vi "StopDrive.vi"(8 "Drive Params":T1={"Omni"=TRUE, "Low Gear"=TRUE}) -> ()   [LabVIEW 2013]
uses:
  AutoDriveParams.ctl
  Drivetrain/Drivetrain Control.ctl
  Drivetrain/DT Mode.ctl
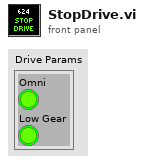
[diagram p1: front panel]
types:
  T1 = typedef "AutoDriveParams.ctl" = cluster{"Omni":bool, "Low Gear":bool}
  T2 = typedef "Drivetrain Control.ctl" = cluster{"axis 1 (x)":dbl, "axis 2 (y)":dbl, "Mode":T3, "heading target":dbl, "steer axis":dbl, "omni?":bool, "Low Gear?":bool, "distance target":cluster{"x":dbl, "y":dbl}, "PID Params":cluster{"X Dist":cluster{"PID gains":cluster{"proportional gain (Kc)":dbl, "integral time (Ti, min)":dbl, "derivative time (Td, min)":dbl}, "output range":cluster{"output high":dbl, "output low":dbl}}, "Y Dist":cluster{"PID gains":cluster{"proportional gain (Kc)":dbl, "integral time (Ti, min)":dbl, "derivative time (Td, min)":dbl}, "output range":cluster{"output high":dbl, "output low":dbl}}}, "Coast":bool}
  T3 = typedef "DT Mode.ctl" = enum16{"Manual", "Gyro Steer", "Distance Drive", "Fieldcentric", "Roll Maneuver", "Alt Roll Maneuver"}
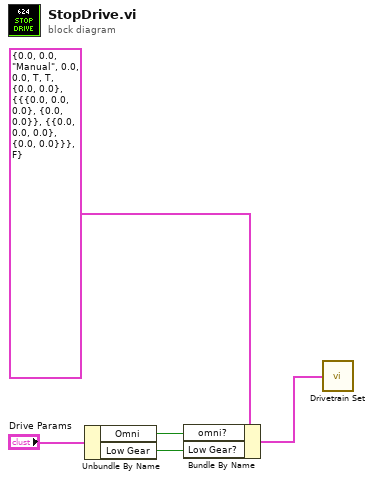
[diagram p0: block diagram]
diagram:
  n1 = Unbundle By Name("Drive Params") -> ("Omni"=w2:bool, "Low Gear"=w1:bool)
  n2 = Bundle By Name(cluster=T2 {"axis 1 (x)"=0.0, "axis 2 (y)"=0.0, "Mode"=enum."Manual", "heading target"=0.0, "steer axis"=0.0, "omni?"=TRUE, "Low Gear?"=TRUE, "distance target"={"x"=0.0, "y"=0.0}, "PID Params"={"X Dist"={"PID gains"={"proportional gain (Kc)"=0.0, "integral time (Ti, min)"=0.0, "derivative time (Td, min)"=0.0}, "output range"={"output high"=0.0, "output low"=0.0}}, "Y Dist"={"PID gains"={"proportional gain (Kc)"=0.0, "integral time (Ti, min)"=0.0, "derivative time (Td, min)"=0.0}, "output range"={"output high"=0.0, "output low"=0.0}}}, "Coast"=FALSE} ("Drivetrain Control"), "omni?"=w2, "Low Gear?"=w1) -> (w3:T2)
  n3 = call "Drivetrain Set.vi"("Drivetrain Control"=w3) -> ()  [unwired: 1 in]
